vi "Determine Warning Good One.vi"(6 "High Wind Speed":dbl, 7 "Current Wind Speed":dbl, 8 "error in (no error)":errorcluster, 9 "Low Temp":dbl, 10 "High Temp":dbl, 11 "Current Temperature":dbl) -> (0 "error out":errorcluster, 1 "Warning?":bool, 2 "Warning Text":string)   [LabVIEW 2010]
doc: "This VI is one solution to an exercise in the LabVIEW Core II course. In this exercise, you take inherited code and improve it for readability and maintainability."
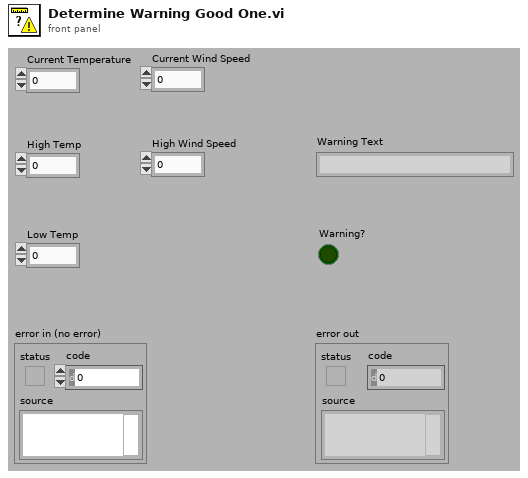
[diagram p1: front panel]
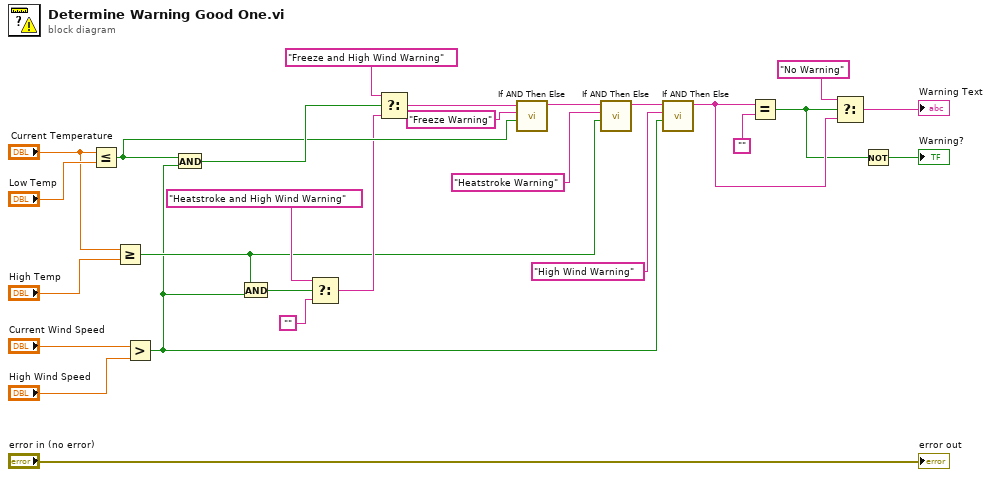
[diagram p0: block diagram]
diagram:
  n1 = Less Or Equal?(x="Current Temperature", y="Low Temp") -> (x <= y?=w17:bool)
  n2 = Greater Or Equal?(x="Current Temperature", y="High Temp") -> (x >= y?=w6:bool)
  n3 = Greater?(x="Current Wind Speed", y="High Wind Speed") -> (0:w3:bool)
  n4 = And(x=w17, y=w3) -> (x .and. y?=w18:bool)
  n5 = And(x=w6, y=w3) -> (x .and. y?=w21:bool)
  n6 = Select(t="Heatstroke and High Wind Warning", s=w21, f="") -> (s? t:f=w15:string)
  n7 = Select(t="Freeze and High Wind Warning", s=w18, f=w15) -> (s? t:f=w10:string)
  n8 = call "If AND Then Else.vi"("AND Condition"=w17, "AND Conditional Text"="Freeze Warning", "Current Text"=w10) -> ("Current Text Out"=w7:string)  [unwired: 6 in]
  n9 = call "If AND Then Else.vi"("AND Condition"=w6, "AND Conditional Text"="Heatstroke Warning", "Current Text"=w7) -> ("Current Text Out"=w4:string)  [unwired: 6 in]
  n10 = call "If AND Then Else.vi"("AND Condition"=w3, "AND Conditional Text"="High Wind Warning", "Current Text"=w4) -> ("Current Text Out"=w2:string)  [unwired: 6 in]
  n11 = Equal?(x=w2, y="") -> (x = y?=w1:bool)
  n12 = Select(t="No Warning" ("f"), s=w1, f=w2) -> (s? t:f=→"Warning Text":string)
  n13 = Not(x=w1) -> (.not. x?=→"Warning?":bool)
  "error out" <- "error in (no error)"
